vi "Dual Etalon Scanner.vi"() -> ()   [LabVIEW 2013]
uses:
  Custom Controls/Dual Etalon LTR Scanner States.ctl
  Global Variables/Global Stop.vi
panel:
  out "back steps":dbl
  out "near the end":bool
  out "Thick Movement Delay":u32
  out "Thin Ready":bool
  out "Thick Ready":bool
  out "Thin has moved":bool
  out "Thick has moved":bool
  out "Loop Counter":i32
  in  "Minimum Stepping Speed [ms]":u32=10
  in  "Tab Control":T1(tab)
  out "Wavenumber Map":dbl[][](graph)
  out "Power Map":dbl[][](graph)
  out "Linewidth Map":dbl[][](graph)
  in  "Stop":bool
  in  "Thin Etalon Position Setpoint":dbl
  in  "Thick Etalon Position Setpoint":dbl
  in  "Scan":bool
  out "Problem":bool
  out "Problem counter":dbl
  out "Thick Etalon Position":dbl
  out "Thin Etalon Position":dbl
  out "row index":dbl
  out "column index":dbl
  in  "Scan Grid Resolution Thin":dbl=20.0
  in  "Scan Grid Size Thick":i32=200
  in  "Scan Grid Size Thin":i32=500
  in  "Scan Grid Resolution Thick":dbl=15.0
  out "WS7 Ch1 Linewidth":dbl format="%.2f"
  out "MPM Ch7 Reference Power":dbl format="%.3p"
  out "WS7 Ch1 Wavenumber":dbl format="%.4f"
  # "To define a new range\nthe Program has to be\nstopped first!"
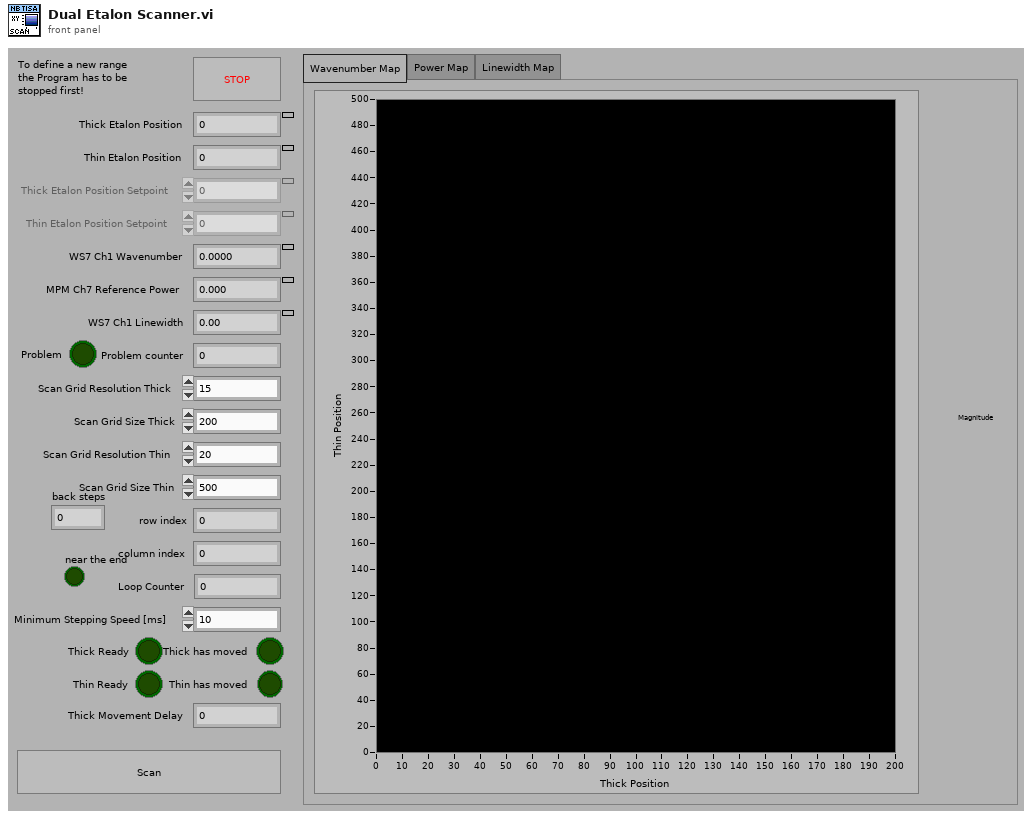
[diagram p1: front panel]
types:
  T1 = enum32{"Wavenumber Map", "Power Map", "Linewidth Map"}
  T2 = typedef "Dual Etalon LTR Scanner States.ctl" = enum16{"Thick Scan", "Thin up", "Thick Reset", "Done"}
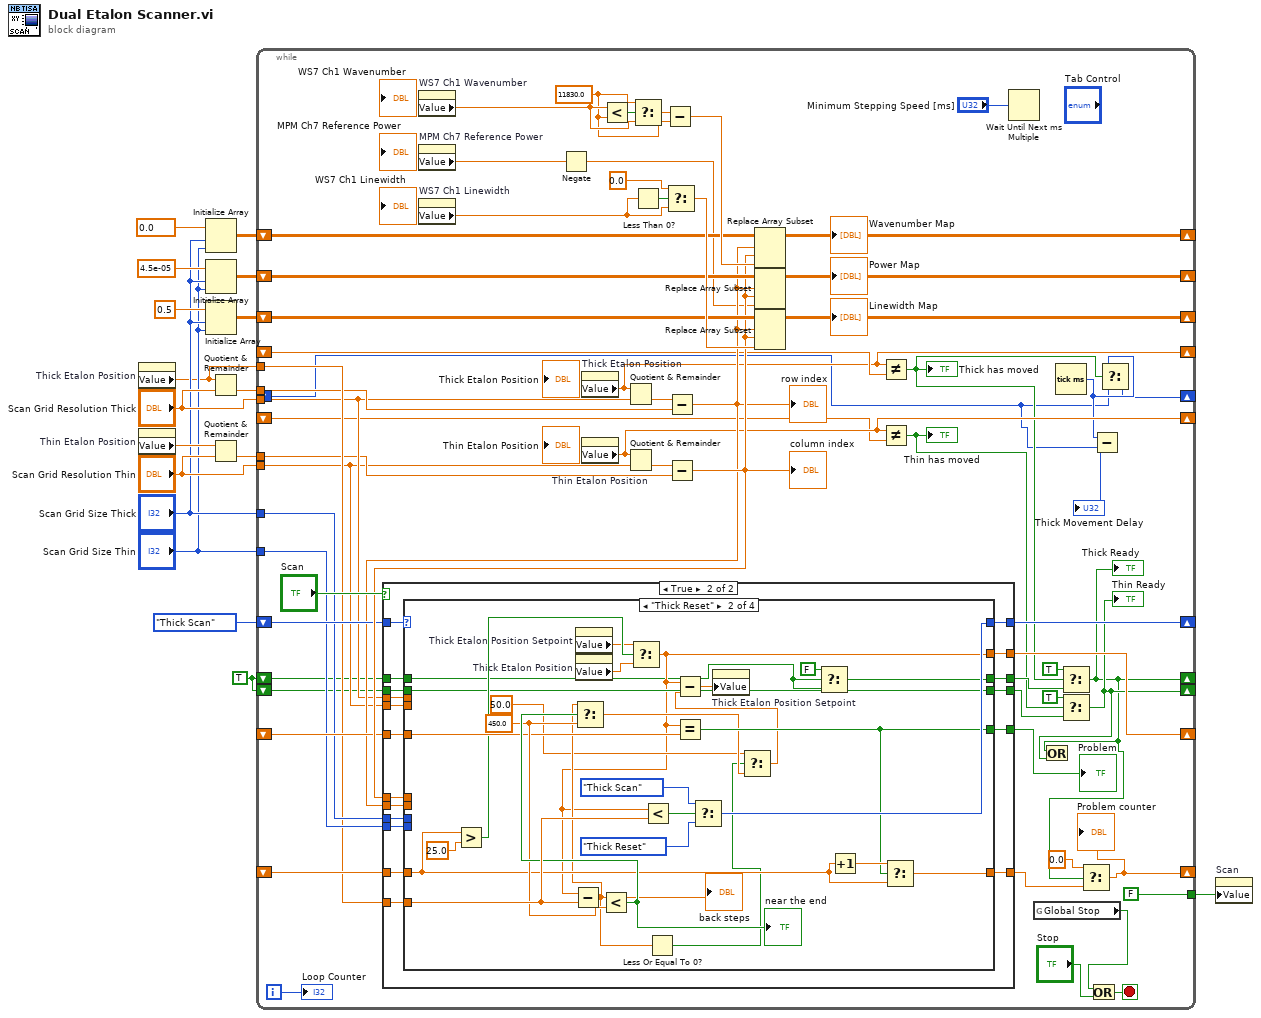
[diagram p0: block diagram]
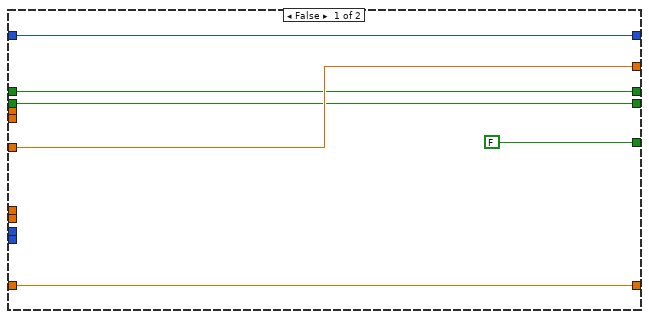
[diagram p2: hidden frame]
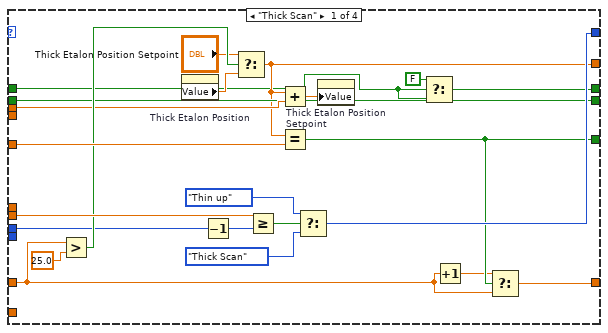
[diagram p3: hidden frame]
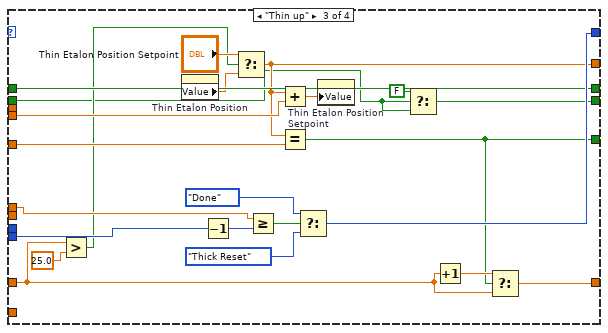
[diagram p4: hidden frame]
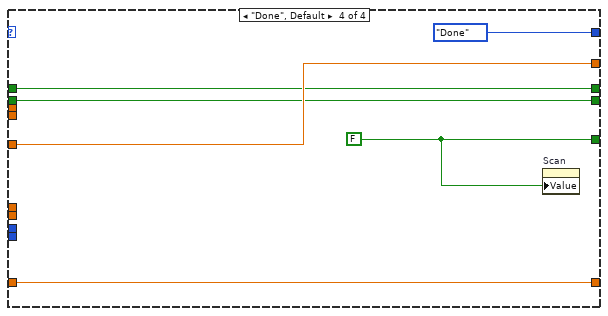
[diagram p5: hidden frame]
diagram:
  w2 = TRUE
  n1 = property on="Thick Etalon Position" class="DigNum (strict)"() -> ("Value"=w3:dbl)  [unwired: 2 in, 2 out]
  n2 = property on="Thin Etalon Position" class="DigNum (strict)"() -> ("Value"=w11:dbl)  [unwired: 2 in, 2 out]
  n3 = Initialize Array(0.0 ("element"), "Scan Grid Size Thick", "Scan Grid Size Thin") -> (w14:dbl[][])
  n4 = Initialize Array(4.5e-05 ("element"), "Scan Grid Size Thick", "Scan Grid Size Thin") -> (w13:dbl[][])
  n5 = Initialize Array(0.5 ("element"), "Scan Grid Size Thick", "Scan Grid Size Thin") -> (w12:dbl[][])
  n6 = Quotient & Remainder(x=w3, y="Scan Grid Resolution Thick") -> (floor(x/y)=w8:dbl)  [unwired: 1 out]
  n7 = Quotient & Remainder(x=w11, y="Scan Grid Resolution Thin") -> (floor(x/y)=w7:dbl)  [unwired: 1 out]
  n8 = while {
    shift-right: [w69] -> _
    shift-left: w14 -> [w72]
    shift-right: [w68] -> _
    shift-left: w13 -> [w71]
    shift-right: [w67] -> _
    shift-left: w12 -> [w70]
    tunnel: "Scan Grid Resolution Thick" -> [w43]
    tunnel: "Scan Grid Resolution Thin" -> [w41]
    tunnel: w8 -> [w44]
    tunnel: w7 -> [w42]
    tunnel: "Scan Grid Size Thick" -> [w53]
    tunnel: "Scan Grid Size Thin" -> [w52]
    shift-right: [w57] -> _
    shift-left: Dual_Etalon_LTR_Scanner_States."Thick Scan" ("Dual Etalon LTR Scanner States") -> [w58]
    shift-right: [w56] -> _
    shift-left: _ -> [w55]
    shift-right: [w25] -> _
    shift-left: _ -> [w51]
    tunnel: w3 -> [w50]
    shift-right: [w39] -> _
    shift-left: _ -> [w40]
    shift-right: [w38] -> _
    shift-left: _ -> [w37]
    shift-right: [w24] -> _
    shift-left: w2 -> [w36]
    shift-right: [w26] -> _
    shift-left: w2 -> [w33]
    tunnel: [FALSE ("Scan")] -> w1
    shift-right: [w21] -> _
    shift-left: _ -> [w20]
    i -> [w48]
    stop <- w45 stop-if-true
    w64 = 11830.0
    n9 = property on="WS7 Ch1 Wavenumber" class="DigNum (strict)"() -> ("Value"=w65:dbl)  [unwired: 2 in, 2 out]
    n10 = property on="MPM Ch7 Reference Power" class="DigNum (strict)"() -> ("Value"=w62:dbl)  [unwired: 2 in, 2 out]
    n11 = property on="WS7 Ch1 Linewidth" class="DigNum (strict)"() -> ("Value"=w66:dbl)  [unwired: 2 in, 2 out]
    n12 = Negate(x=w62) -> (-x=w18:dbl)
    n13 = property on="Thick Etalon Position" class="DigNum (strict)"() -> ("Value"=w39:dbl)  [unwired: 2 in, 2 out]
    n14 = property on="Thin Etalon Position" class="DigNum (strict)"() -> ("Value"=w38:dbl)  [unwired: 2 in, 2 out]
    n15 = Less?(x=w65, y=w64) -> (x < y?=w73:bool)
    n16 = Quotient & Remainder(x=w39, y=w43) -> (floor(x/y)=w74:dbl)  [unwired: 1 out]
    n17 = Quotient & Remainder(x=w38, y=w41) -> (floor(x/y)=w75:dbl)  [unwired: 1 out]
    n18 = Select(t=w64, s=w73, f=w65) -> (s? t:f=w63:dbl)
    n19 = Less Than 0?(x=w66) -> (x < 0?=w76:bool)
    n20 = Subtract(x=w63, y=w64) -> (x-y=w79:dbl)
    n21 = Select(t=0.0, s=w76, f=w66) -> (s? t:f=w78:dbl)
    n22 = Subtract(x=w74, y=w44) -> (x-y=w54:dbl)
    "row index" <- w54
    n23 = Subtract(x=w75, y=w42) -> (x-y=w59:dbl)
    "column index" <- w59
    n24 = case shown="True" "Scan" {
      tunnel: w58 -> [w85 w102]
      tunnel: [w85 w103] -> w57
      tunnel: w41 -> [_ w101]
      tunnel: w53 -> [_ w100]
      tunnel: w54 -> [_ w99]
      tunnel: w59 -> [_ w98]
      tunnel: w50 -> [_ w97]
      tunnel: w55 -> [w84 w96]
      tunnel: [w84 w95] -> w56
      tunnel: [FALSE w94] -> w61
      tunnel: w51 -> [w82 w93]
      tunnel: [w82 w92] -> w27
      tunnel: w52 -> [_ w91]
      tunnel: w43 -> [_ w90]
      tunnel: [w81 w89] -> w34
      tunnel: w36 -> [w81 w88]
      tunnel: w33 -> [w80 w87]
      tunnel: [w80 w86] -> w30
      frame False {
      }
      frame True {
        n25 = case shown="\"Thick Reset\"" w102 {
          tunnel: [w122 w151 w171 Dual_Etalon_LTR_Scanner_States."Done" ("Dual Etalon LTR Scanner States")] -> w103
          tunnel: w101 -> [_ _ w176 _]
          tunnel: w100 -> [w117 _ _ _]
          tunnel: w99 -> [w121 _ _ _]
          tunnel: w98 -> [_ _ w170 _]
          tunnel: w97 -> [_ w149 _ _]
          tunnel: w96 -> [w120 w146 w169 w181]
          tunnel: [w107 w130 w157 w181] -> w95
          tunnel: [w111 w136 w160 w179] -> w94
          tunnel: w93 -> [w109 w137 w161 w180]
          tunnel: [w108 w138 w162 w180] -> w92
          tunnel: w91 -> [_ _ w168 _]
          tunnel: w90 -> [w116 _ _ _]
          tunnel: [w105 w128 w165 w178] -> w89
          tunnel: w88 -> [w104 w127 w165 w178]
          tunnel: w87 -> [w112 w140 w154 w177]
          tunnel: [w112 w140 w155 w177] -> w86
          frame "Thick Scan" {
            n26 = Greater?(x=w109, y=25.0) -> (0:w118:bool)
            n27 = property on="Thick Etalon Position" class="DigNum (strict)"() -> ("Value"=w113:dbl)  [unwired: 2 in, 2 out]
            n28 = Decrement(x=w117) -> (x-1=w125:i32)
            n29 = Select(t="Thick Etalon Position Setpoint", s=w118, f=w113) -> (s? t:f=w107:dbl)
            n30 = Greater Or Equal?(x=w121, y=w125) -> (x >= y?=w126:bool)
            n31 = Add(x=w107, y=w116) -> (x+y=w115:dbl)
            n32 = Equal?(x=w107, y=w120) -> (x = y?=w111:bool)
            n33 = Select(t=Dual_Etalon_LTR_Scanner_States."Thin up" ("Dual Etalon LTR Scanner States"), s=w126, f=Dual_Etalon_LTR_Scanner_States."Thick Scan" ("Dual Etalon LTR Scanner States")) -> (s? t:f=w122:T2)
            n34 = property on="Thick Etalon Position Setpoint" class="DigNum (strict)"("Value"=w115) -> ()  [unwired: 2 in, 2 out]
            n35 = Select(t=FALSE, s=w104, f=w104) -> (s? t:f=w105:bool)
            n36 = Increment(x=w109) -> (x+1=w110:dbl)
            n37 = Select(t=w110, s=w111, f=w109) -> (s? t:f=w108:dbl)
          }
          frame "Thick Reset" {
            w147 = 450.0 ("y")
            n38 = Greater?(x=w137, y=25.0) -> (0:w144:bool)
            n39 = property on="Thick Etalon Position Setpoint" class="DigNum (strict)"() -> ("Value"=w142:dbl)  [unwired: 2 in, 2 out]
            n40 = property on="Thick Etalon Position" class="DigNum (strict)"() -> ("Value"=w141:dbl)  [unwired: 2 in, 2 out]
            n41 = Select(t=w142, s=w144, f=w141) -> (s? t:f=w130:dbl)
            n42 = Subtract(x=w130, y=w149) -> (x-y=w135:dbl)
            "back steps" <- w135
            n43 = Less?(x=w135, y=w147) -> (x < y?=w148:bool)
            "near the end" <- w148
            n44 = Select(t=w135, s=w148, f=w147) -> (s? t:f=w134:dbl)
            n45 = Less?(x=w130, y=w149) -> (x < y?=w150:bool)
            n46 = Less Or Equal To 0?(x=w135) -> (x <= 0?=w132:bool)
            n47 = Equal?(x=w130, y=w146) -> (x = y?=w136:bool)
            n48 = Select(t=Dual_Etalon_LTR_Scanner_States."Thick Scan" ("Dual Etalon LTR Scanner States"), s=w150, f=Dual_Etalon_LTR_Scanner_States."Thick Reset" ("Dual Etalon LTR Scanner States")) -> (s? t:f=w151:T2)
            n49 = Select(t=50.0 ("y"), s=w132, f=w134) -> (s? t:f=w133:dbl)
            n50 = Subtract(x=w130, y=w133) -> (x-y=w143:dbl)
            n51 = property on="Thick Etalon Position Setpoint" class="DigNum (strict)"("Value"=w143) -> ()  [unwired: 2 in, 2 out]
            n52 = Select(t=FALSE, s=w127, f=w127) -> (s? t:f=w128:bool)
            n53 = Increment(x=w137) -> (x+1=w139:dbl)
            n54 = Select(t=w139, s=w136, f=w137) -> (s? t:f=w138:dbl)
          }
          frame "Thin up" {
            n55 = Greater?(x=w161, y=25.0) -> (0:w159:bool)
            n56 = property on="Thin Etalon Position" class="DigNum (strict)"() -> ("Value"=w158:dbl)  [unwired: 2 in, 2 out]
            n57 = Decrement(x=w168) -> (x-1=w174:i32)
            n58 = Select(t="Thin Etalon Position Setpoint", s=w159, f=w158) -> (s? t:f=w157:dbl)
            n59 = Greater Or Equal?(x=w170, y=w174) -> (x >= y?=w175:bool)
            n60 = Add(x=w157, y=w176) -> (x+y=w167:dbl)
            n61 = Equal?(x=w157, y=w169) -> (x = y?=w160:bool)
            n62 = Select(t=Dual_Etalon_LTR_Scanner_States."Done" ("Dual Etalon LTR Scanner States"), s=w175, f=Dual_Etalon_LTR_Scanner_States."Thick Reset" ("Dual Etalon LTR Scanner States")) -> (s? t:f=w171:T2)
            n63 = property on="Thin Etalon Position Setpoint" class="DigNum (strict)"("Value"=w167) -> ()  [unwired: 2 in, 2 out]
            n64 = Select(t=FALSE, s=w154, f=w154) -> (s? t:f=w155:bool)
            n65 = Increment(x=w161) -> (x+1=w163:dbl)
            n66 = Select(t=w163, s=w160, f=w161) -> (s? t:f=w162:dbl)
          }
          frame "Done", Default {
            w179 = FALSE
            n67 = property on="Scan" class="Bool (strict)"("Value"=w179) -> ()  [unwired: 2 in, 2 out]
          }
        }
      }
    }
    "Problem" <- w61
    n68 = Replace Array Subset(array=w72, new element=w79, index (row)=w54, index (col)=w59) -> (w69:dbl[][])
    "Wavenumber Map" <- w69
    n69 = Replace Array Subset(array=w71, new element=w18, index (row)=w54, index (col)=w59) -> (w68:dbl[][])
    "Power Map" <- w68
    n70 = Replace Array Subset(array=w70, new element=w78, index (row)=w54, index (col)=w59) -> (w67:dbl[][])
    "Linewidth Map" <- w67
    n71 = Not Equal?(x=w39, y=w40) -> (x != y?=w23:bool)
    "Thick has moved" <- w23
    n72 = Not Equal?(x=w38, y=w37) -> (x != y?=w31:bool)
    "Thin has moved" <- w31
    n73 = Wait Until Next ms Multiple(millisecond multiple="Minimum Stepping Speed [ms]") -> ()  [unwired: 1 out]
    n74 = global read "Global Stop.vi" "Global Stop"() -> (w46:bool)
    n75 = Tick Count (ms)() -> (millisecond timer value=w22:u32)
    n76 = Select(t=TRUE, s=w23, f=w34) -> (s? t:f=w24:bool)
    "Thick Ready" <- w24
    n77 = Select(t=TRUE, s=w31, f=w30) -> (s? t:f=w26:bool)
    "Thin Ready" <- w26
    n78 = Or(x=w24, y=w26) -> ()  [unwired: 1 out]
    n79 = Select(t=0.0, s=w24, f=w27) -> (s? t:f=w25:dbl)
    "Problem counter" <- w25
    n80 = Or(x=w46, y="Stop") -> (x .or. y?=w45:bool)
    n81 = Subtract(x=w22, y=w20) -> (x-y=→"Thick Movement Delay":u32)
    n82 = Select(t=w22, s=w23, f=w20) -> (s? t:f=w21:u32)
    "Loop Counter" <- w48
  }
  n83 = property on="Scan" class="Bool (strict)"("Value"=w1) -> ()  [unwired: 2 in, 2 out]
